vi "New Waveform Stream Specification.vi"(8 "error in (no error)":errorcluster, 11 "waveform path":string) -> (0 "error out":errorcluster, 3 "WaveformStreamSpecification":T1)   [LabVIEW 2020, in "NI_VS Waveform Streaming Interface.lvlib"]
doc: "Identifies a waveform whose data you want to stream to a host computer."
uses:
  <vilib>/NI VeriStand/Execution/WaveformStreaming/NI_VS Waveform Streaming Interface.lvlib
  <vilib>/NI VeriStand/Execution/WaveformStreaming/WaveformStreamSpecification.ctl
  NationalInstruments.VeriStand.ClientAPI
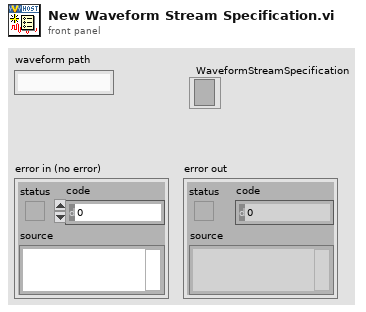
[diagram p1: front panel]
types:
  T1 = typedef "NI_VS Waveform Streaming Interface.lvlib/WaveformStreamSpecification.ctl" = refnum<k24>
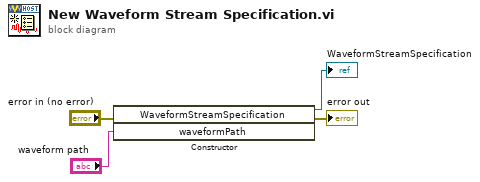
[diagram p0: block diagram]
diagram:
  n1 = constructor class="WaveformStreamSpecification"(error in="error in (no error)", "waveformPath"="waveform path") -> (reference out=→"WaveformStreamSpecification":refnum<k24>, error out=→"error out":errorcluster)  [unwired: 2 in, 2 out]
